vi "Camera Servo Control by Joystick.vi"(9 "axis control":dbl(slide) scale=-1.0..1.0, 10 "max jump angle":i32) -> (3 "angle set":i32)   [LabVIEW 2013]
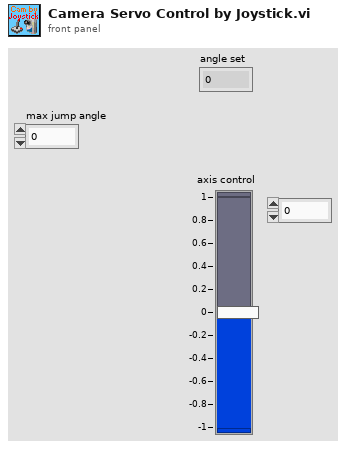
[diagram p1: front panel]
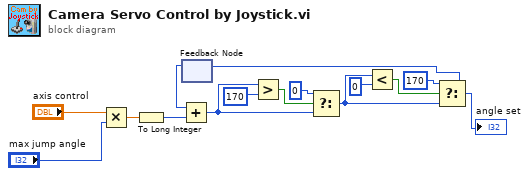
[diagram p0: block diagram]
diagram:
  n1 = Multiply(x="axis control", y="max jump angle") -> (x*y=w10:dbl)
  n2 = To Long Integer(number=w10) -> (32bit integer=w13:i32)
  n3 = feedback #1() -> (w14:i32)  [unwired: 1 in]
  n4 = Add(x=w14, y=w13) -> (x+y=w6:i32)
  n5 = Greater?(x=w6, y=170) -> (0:w7:bool)
  n6 = Select(t=0, s=w7, f=w6) -> (s? t:f=w1:i32)
  n7 = Less?(x=w1, y=0) -> (x < y?=w2:bool)
  n8 = Select(t=170, s=w2, f=w1) -> (s? t:f=w3:i32)
  "angle set" <- w3
  n9 = feedback-in #1(w3) -> ()
